vi "InsetStringToFileGcode.vi"(8 "error in (no error)":errorcluster, 10 "StringFileGcode":string, 11 "ParameterConf in":refnum<class "ParameterConf.lvclass">) -> (0 "error out":errorcluster, 3 "ParameterConf out":refnum<class "ParameterConf.lvclass">)   [LabVIEW 2017, in "LibraryGcode.lvlib" / "ParameterConf.lvclass"]
uses:
  ParameterConf.lvclass
  ParameterConf.lvclass/ParameterConf.ctl
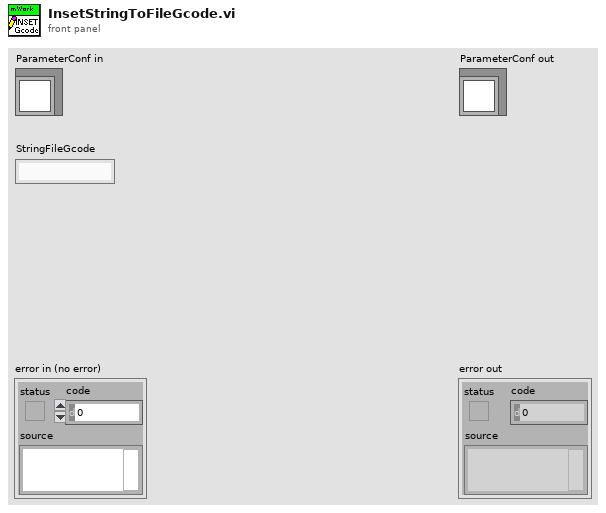
[diagram p1: front panel]
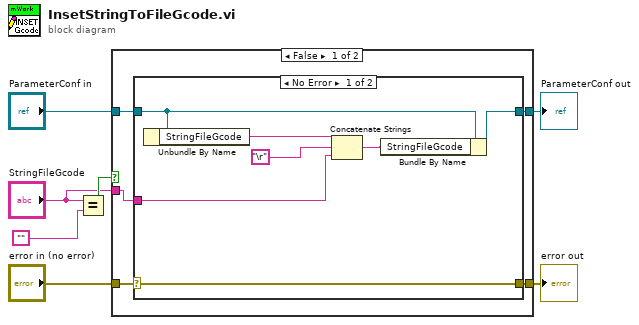
[diagram p0: block diagram]
diagram:
  n1 = Equal?(x="StringFileGcode", y="") -> (x = y?=w2:bool)
  n2 = case shown="False" w2 {
    tunnel: "error in (no error)" -> [w12 w22]
    tunnel: [w11 w22] -> w6
    tunnel: "ParameterConf in" -> [w10 w23]
    tunnel: [w9 w23] -> w4
    tunnel: "StringFileGcode" -> [w8 _]
    frame False {
      n3 = case shown="No Error" w12 {
        selector: w12 -> [w19 w20]
        tunnel: [w19 w20] -> w11
        tunnel: [w18 w21] -> w9
        tunnel: w10 -> [w15 w21]
        tunnel: w8 -> [w17 _]
        frame No Error {
          n4 = Unbundle By Name(w15) -> ("StringFileGcode"=w14:string)
          n5 = Concatenate Strings(w14, "\r", w17) -> (w16:string)
          n6 = Bundle By Name(cluster=w15, "StringFileGcode"=w16) -> (w18:refnum<class "ParameterConf.lvclass">)
        }
        frame Error {
        }
      }
    }
    frame True {
    }
  }
  "error out" <- w6
  "ParameterConf out" <- w4
